vi "Media Player Example.vi"() -> ()   [LabVIEW 2020]
doc: "Simple example of audio device playback of a file decoded with G-Audio."
uses:
  Audio Files/Polymorphic VIs/Get Audio File Info (Path).vi
  Private/Path To UTF-8 String.vi
  Audio Files/Private/Get Audio File Info (Core).vi
  Private/Result To Error.vi
  <vilib>/Utility/error.llb/Error Cluster From Error Code.vi
  G-Audio.lvlib
panel:
  in  "Playlist":i32(listbox)
  out "error out":errorcluster
  # "G"
  # "-Audio"
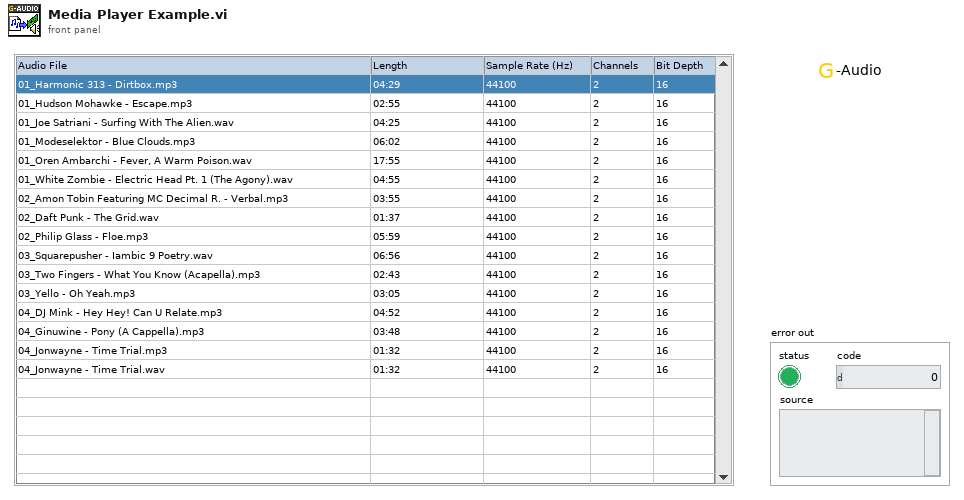
[diagram p1: front panel]
types:
  T1 = typedef "G-Audio.lvlib/Audio File Info.ctl" = cluster{"Sample Rate (Hz)":u32, "Channels":u32, "Bit Depth":u32}
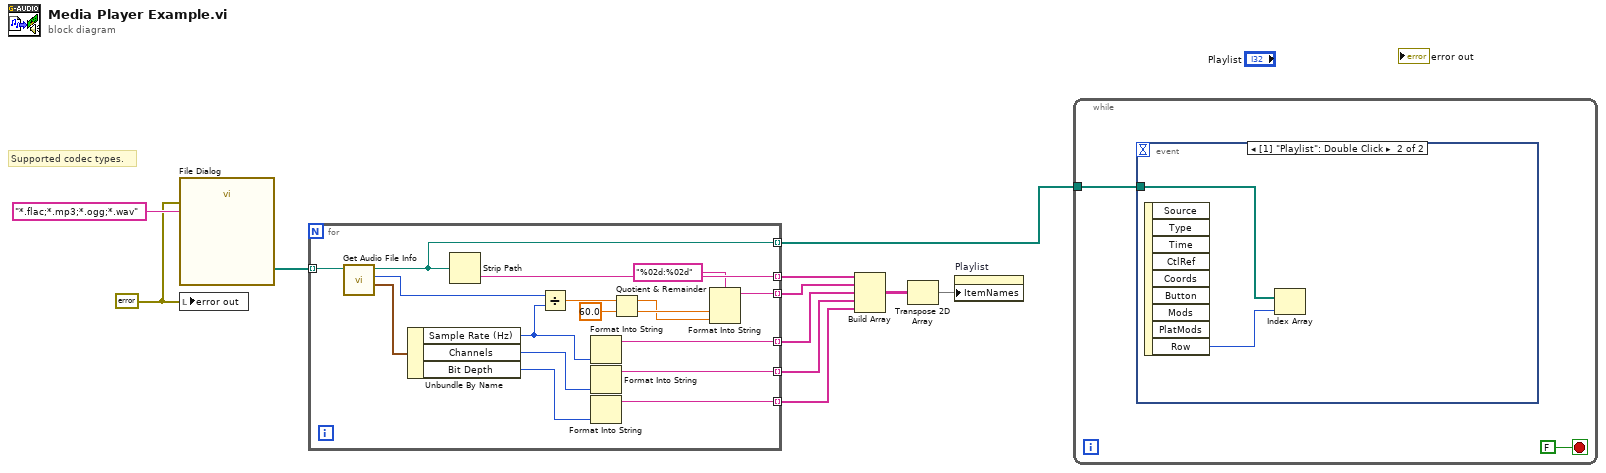
[diagram p0: block diagram]
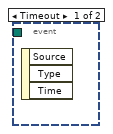
[diagram p2: hidden frame]
diagram:
  w10 = errorcluster {"status"=FALSE, "code"=0, "source"=""} ("error out")
  # "Supported codec types."
  n1 = call "File Dialog"("error in"=w10, "pattern (all files)"="*.flac;*.mp3;*.ogg;*.wav") -> ("selected paths"=w9:path[])  [unwired: 10 in, 3 out]
  n2 = local write "error out"(w10) -> ()
  n3 = for {
    tunnel: w9 -> [w28] mode=indexing
    tunnel: [w27] -> w7 mode=indexing
    tunnel: [w23] -> w5 mode=indexing
    tunnel: [w20] -> w4 mode=indexing
    tunnel: [w19] -> w3 mode=indexing
    tunnel: [w13] -> w2 mode=indexing
    tunnel: [w12] -> w1 mode=indexing
    n4 = call-poly "Get Audio File Info.vi"("Path In"=w28) -> ("Audio File Info"=w26:T1, "PCM Frame Length"=w25:u64, "Path Out"=w12:path)  [unwired: 6 in, 2 out]
    n5 = Unbundle By Name(w26) -> ("Sample Rate (Hz)"=w24:u32, "Channels"=w22:u32, "Bit Depth"=w21:u32)
    n6 = Strip Path(path=w12) -> (name=w27:string)  [unwired: 1 out]
    n7 = Divide(x=w25, y=w24) -> (x/y=w18:dbl)
    n8 = Format Into String(w24) -> (resulting string=w23:string)  [unwired: 3 in, 1 out]
    n9 = Format Into String(w22) -> (resulting string=w20:string)  [unwired: 3 in, 1 out]
    n10 = Format Into String(w21) -> (resulting string=w19:string)  [unwired: 3 in, 1 out]
    n11 = Quotient & Remainder(x=w18, y=60.0) -> (x-y*floor(x/y)=w14:dbl, floor(x/y)=w15:dbl)
    n12 = Format Into String(format string="%02d:%02d", w15, w14) -> (resulting string=w13:string)  [unwired: 2 in, 1 out]
  }
  n13 = Build Array(w7, w2, w5, w4, w3) -> (w8:string[][])
  n14 = Transpose 2D Array(2D array=w8) -> (transposed array=w6:string[][])
  n15 = property on="Playlist" class="MCListbox (strict)"("ItemNames"=w6) -> ()  [unwired: 2 in, 2 out]
  n16 = while {
    tunnel: w1 -> [w30]
    stop <- FALSE stop-if-true
    n17 = event shown="[1] \"Playlist\": Double Click" {
      selector: _ -> [_ _]
      dyn-events: _ -> [_ _]
      timeout: _ -> [_ _]
      tunnel: w30 -> [_ w32]
      event Timeout {
        n18 = event-data() -> ()  [unwired: 1 in, 3 out]
      }
      event "Playlist": Double Click {
        n19 = event-data() -> ("Row"=w31:i32)  [unwired: 1 in, 8 out]
        n20 = Index Array(array=w32, index=w31) -> ()  [unwired: 1 out]
      }
    }
  }
